vi "Invalid Application Refnum.vi"() -> ()   [LabVIEW 2017, in "Assertion.Tests.lvlib" / "Assert Not Refnum.lvlib"]
uses:
  Assert Not Refnum.lvlib
  Assertion/Assertion.lvlib
panel:
  out "error out":errorcluster
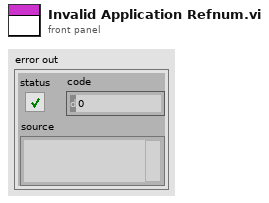
[diagram p1: front panel]
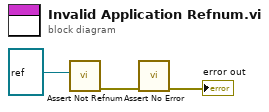
[diagram p0: block diagram]
diagram:
  n1 = call "Assert Not Refnum.vi"("Refnum"=refnum<vi> refnum ("App Refnum")) -> ("error out"=w3:errorcluster)  [unwired: 10 in]
  n2 = call "Assert No Error.vi"("error in (no error)"=w3) -> ("error out"=→"error out":errorcluster)  [unwired: 10 in]
